vi "Databasetesting.vi"() -> ()   [LabVIEW 2020]
uses:
  Database/Control 1.ctl
  <vilib>/addons/database/Connection.llb/DB Tools Open Connec (Path).vi
  <vilib>/addons/database/_DB Variant To Data/Database Variant To Data.xnode
  <vilib>/addons/database/NI_Database_API.lvlib
panel:
  out "x = y?":bool
  out "number":i32
  out "ID 2":i32 min=0
  in  "stop":bool
  in  "connection information":path=path "C:/Users/User/Documents/Database/Database.udl"
  in  "Tab Control":T1(tab)
  out "Data in Database":string[][][](array[string])
  in  "ID":i32 min=0
  in  "Delete Student":bool
  in  "Add Student":bool
  in  "Add Student Parameters":T2
  in  "Listbox":i32(listbox)
  out "Manipulate Array":string[][](array[string])
  out "Row to Delete":string[][](array[string])
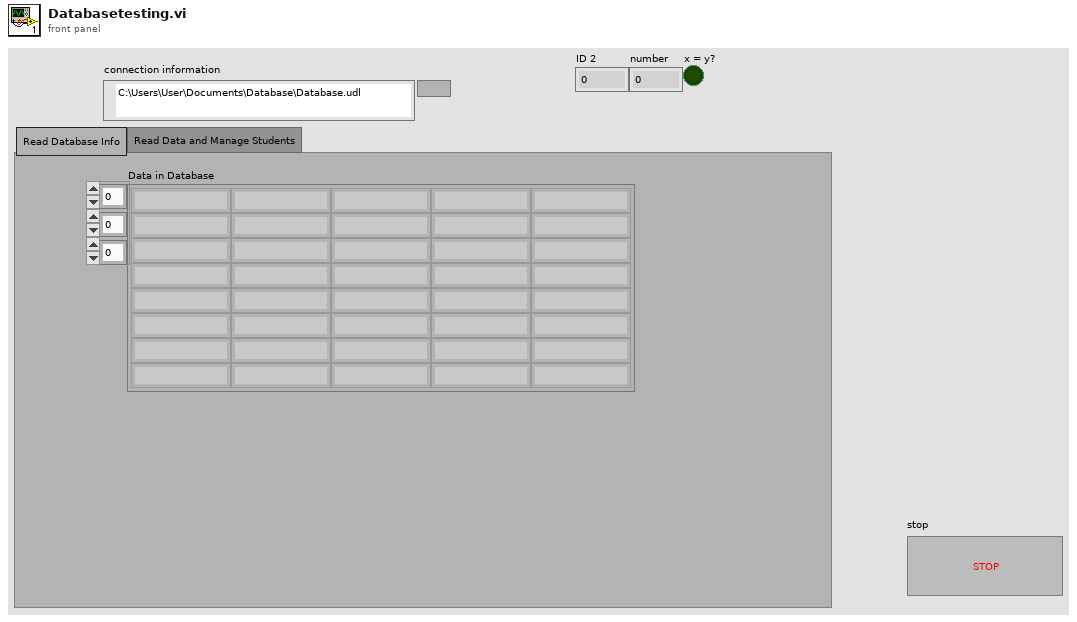
[diagram p1: front panel]
types:
  T1 = enum32{"Read Database Info", "Read Data and Manage Students"}
  T2 = cluster{"Credit Hours":dbl, "Name":string, "Major":string, "Class Rank":string, "ID":i32}
  T3 = typedef "Control 1.ctl" = enum16{"Init Read", "Init Manipulate", "Wait for GUI", "Add Student", "Delete Student", "Stop"}
  T4 = typedef "NI_Database_API.lvlib/Conn ObjectReference.ctl" = refnum<k1>
  T5 = typedef "NI_Database_API.lvlib/DB Tools DataTypes.ctl" = enum16{"String", "Long (I32)", "Single (SGL)", "Double (DBL)", "Date/Time", "Binary"}
  T6 = cluster{"name":string, "database data type":T5, "defined size":i32}[]
  T7 = cluster{"ID":i32, "Name":string, "Major":string, "Credit Hours":dbl, "Class Rank":string}
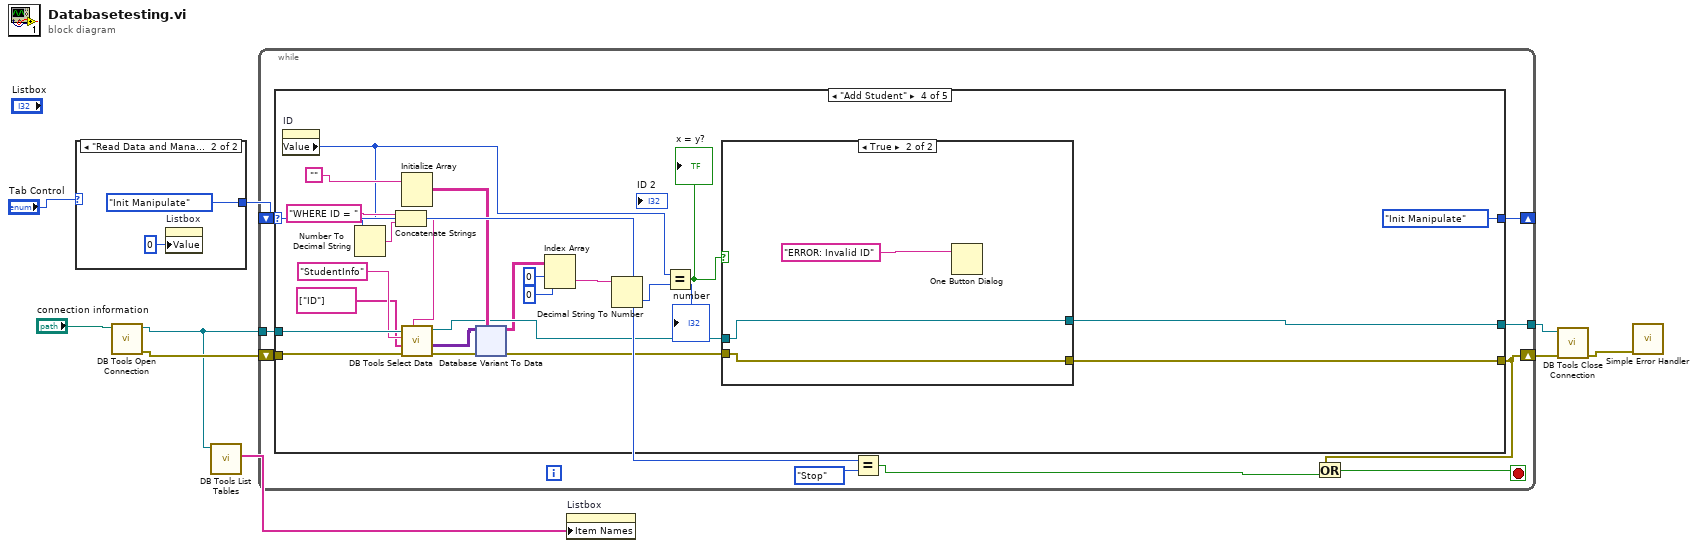
[diagram p0: block diagram]
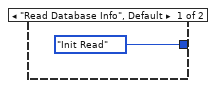
[diagram p2: hidden frame]
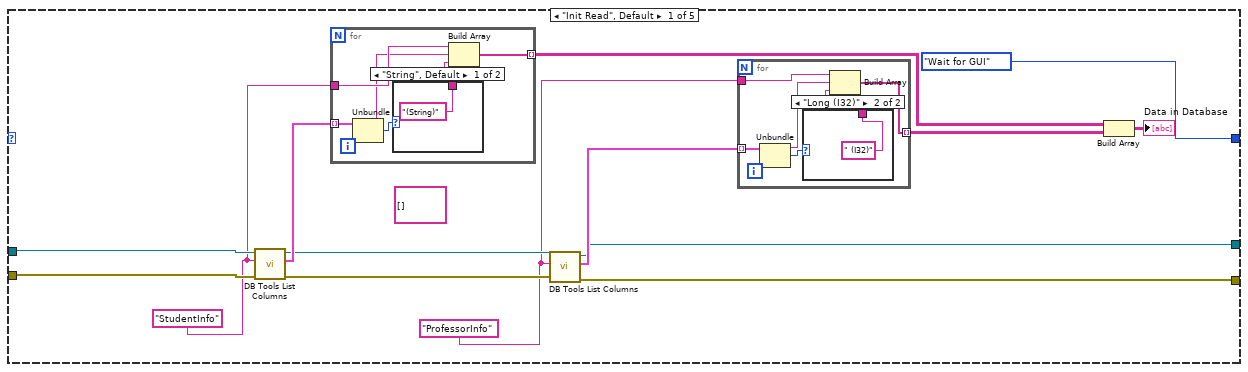
[diagram p3: hidden frame]
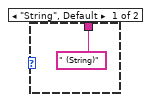
[diagram p4: hidden frame]
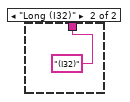
[diagram p5: hidden frame]
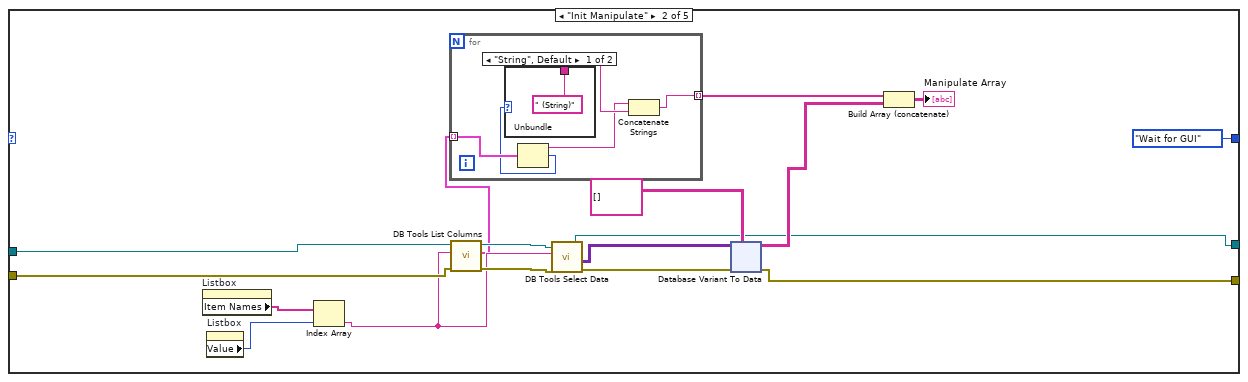
[diagram p6: hidden frame]
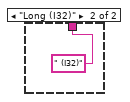
[diagram p7: hidden frame]
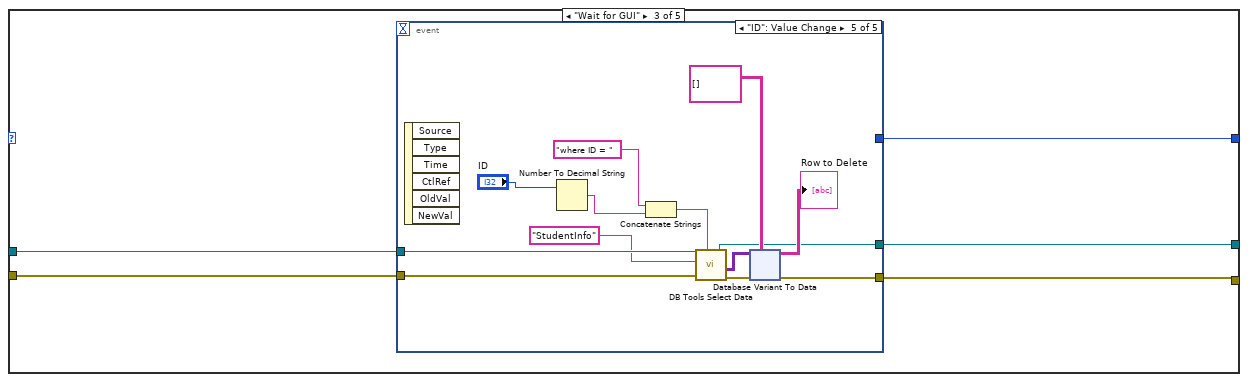
[diagram p8: hidden frame]
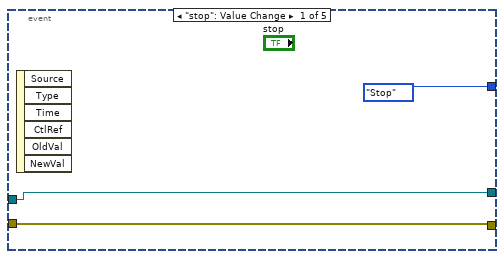
[diagram p9: hidden frame]
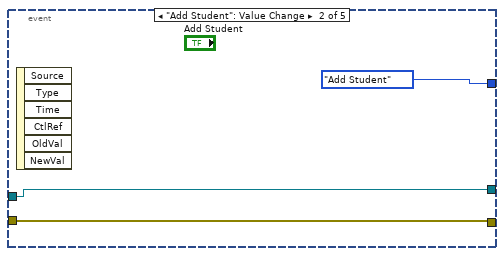
[diagram p10: hidden frame]
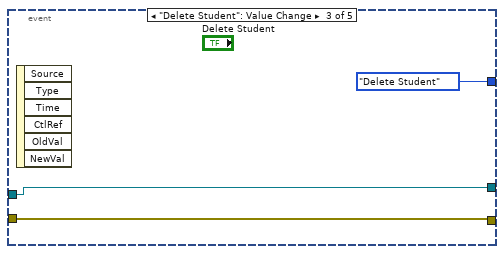
[diagram p11: hidden frame]
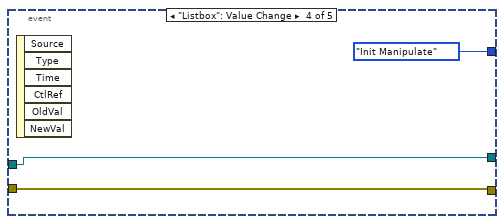
[diagram p12: hidden frame]
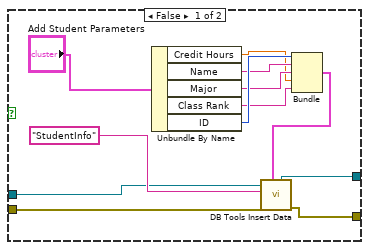
[diagram p13: hidden frame]
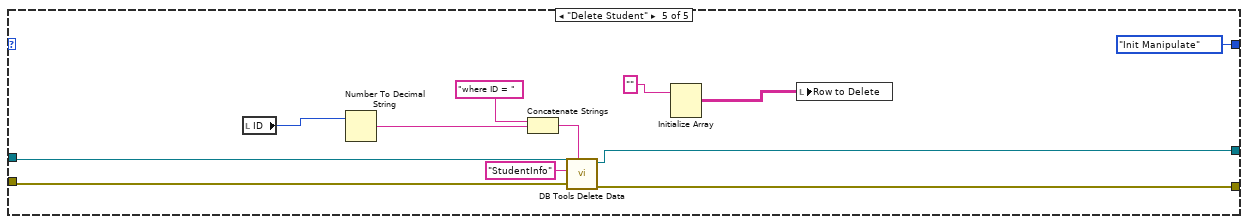
[diagram p14: hidden frame]
diagram:
  n1 = case shown="\"Read Data and Manage Students\"" "Tab Control" {
    tunnel: [Control_1."Init Read" Control_1."Init Manipulate"] -> w7
    frame "Read Database Info", Default {
    }
    frame "Read Data and Manage Students" {
      n2 = property on="Listbox" class="LstBox (strict)"("Value"=0 ("Listbox")) -> ()  [unwired: 2 in, 2 out]
    }
  }
  n3 = call-poly <vilib>:"DB Tools Open Connection.vi"("connection information"="connection information") -> ("error out"=w8:errorcluster, "connection reference"=w6:T4)  [unwired: 7 in]
  n4 = call <vilib>:"DB Tools List Tables.vi"("connection reference"=w6) -> ("tables"=w5:string[])  [unwired: 4 in, 2 out]
  n5 = while {
    tunnel: w6 -> [w19]
    shift-right: [w18] -> _
    shift-left: w7 -> [w21]
    tunnel: [w16] -> w3
    shift-right: [w14] -> w2
    shift-left: w8 -> [w20]
    stop <- w13 stop-if-true
    n6 = case shown="\"Add Student\"" w21 {
      tunnel: w20 -> [w34 w67 w122 w212 w287]
      tunnel: w19 -> [w33 w68 w123 w213 w286]
      tunnel: [Control_1."Wait for GUI" Control_1."Wait for GUI" w124 Control_1."Init Manipulate" Control_1."Init Manipulate"] -> w18
      tunnel: [w28 w54 w121 w216 w285] -> w16
      tunnel: [w27 w53 w120 w214 w284] -> w14
      frame "Init Read", Default {
        w24 = "ProfessorInfo" ("table")
        (unwired) string[][] [] ("initialized array")
        w26 = "StudentInfo" ("table")
        n7 = call <vilib>:"DB Tools List Columns.vi"("error in (no error)"=w34, "table"=w26, "connection reference"=w33) -> ("error out"=w29:errorcluster, "column information"=w32:T6, "connection reference out"=w30:T4)  [unwired: 1 in, 1 out]
        n8 = for {
          tunnel: w32 -> [w49] mode=indexing
          tunnel: w26 -> [w47]
          tunnel: [w44] -> w25 mode=indexing
          n9 = Unbundle(w49) -> ("name"=w46:string, "database data type"=w48:T5)  [unwired: 1 out]
          n10 = case shown="\"String\", Default" w48 {
            tunnel: ["(String)" "(I32)"] -> w45
            frame "String", Default {
            }
            frame "Long (I32)" {
            }
          }
          n11 = Build Array(w47, w46, w45) -> (w44:string[])
        }
        n12 = call <vilib>:"DB Tools List Columns.vi"("error in (no error)"=w29, "table"=w24, "connection reference"=w30) -> ("error out"=w27:errorcluster, "column information"=w31:T6, "connection reference out"=w28:T4)  [unwired: 1 in, 1 out]
        n13 = for {
          tunnel: w31 -> [w41] mode=indexing
          tunnel: w24 -> [w38]
          tunnel: [w36] -> w23 mode=indexing
          n14 = Unbundle(w41) -> ("name"=w39:string, "database data type"=w40:T5)  [unwired: 1 out]
          n15 = case shown="\"Long (I32)\"" w40 {
            tunnel: [" (String)" " (I32)"] -> w37
            frame "String", Default {
            }
            frame "Long (I32)" {
            }
          }
          n16 = Build Array(w38, w39, w37) -> (w36:string[])
        }
        n17 = Build Array(w25, w23) -> (→"Data in Database":string[][][])
      }
      frame "Init Manipulate" {
        n18 = property on="Listbox" class="LstBox (strict)"() -> ("Item Names"=w60:string[])  [unwired: 2 in, 2 out]
        n19 = property on="Listbox" class="LstBox (strict)"() -> ("Value"=w59:i32)  [unwired: 2 in, 2 out]
        n20 = Index Array(array=w60, index=w59) -> (element=w58:string)
        n21 = call <vilib>:"DB Tools List Columns.vi"("error in (no error)"=w67, "table"=w58, "connection reference"=w68) -> ("error out"=w63:errorcluster, "column information"=w57:T6, "connection reference out"=w64:T4)  [unwired: 1 in, 1 out]
        n22 = for {
          tunnel: w57 -> [w73] mode=indexing
          tunnel: [w69] -> w56 mode=indexing
          n23 = Unbundle(w73) -> ("name"=w70:string, "database data type"=w71:T5)  [unwired: 1 out]
          n24 = case shown="\"String\", Default" w71 {
            tunnel: [" (String)" " (I32)"] -> w72
            frame "String", Default {
            }
            frame "Long (I32)" {
            }
          }
          n25 = Concatenate Strings(w70, w72) -> (w69:string)
        }
        n26 = call <vilib>:"DB Tools Select Data.vi"("error in (no error)"=w63, "table"=w58, "connection reference"=w64) -> ("error out"=w65:errorcluster, "data"=w66:variant[][], "connection reference out"=w54:T4)  [unwired: 3 in]
        n27 = xnode "Database Variant To Data"("database variant"=w66, "error in (no error)"=w65, "type"=string[][] [] ("initialized array")) -> ("data"=w61:string[][], "error out"=w53:errorcluster)
        n28 = Build Array (concatenate)(w56, w61) -> (→"Manipulate Array":string[][])
      }
      frame "Wait for GUI" {
        n29 = event shown="[4] \"ID\": Value Change" {
          selector: _ -> [_ _ _ _ _]
          dyn-events: _ -> [_ _ _ _ _]
          timeout: _ -> [_ _ _ _ _]
          tunnel: [Control_1."Stop" Control_1."Add Student" Control_1."Delete Student" Control_1."Init Manipulate" _] -> w124
          tunnel: w123 -> [w126 w129 w132 w135 w148]
          tunnel: w122 -> [w125 w128 w131 w134 w149]
          tunnel: [w126 w129 w132 w135 w137] -> w121
          tunnel: [w125 w128 w131 w134 w138] -> w120
          event "stop": Value Change {
            n30 = event-data() -> ()  [unwired: 1 in, 6 out]
          }
          event "Add Student": Value Change {
            n31 = event-data() -> ()  [unwired: 1 in, 6 out]
          }
          event "Delete Student": Value Change {
            n32 = event-data() -> ()  [unwired: 1 in, 6 out]
          }
          event "Listbox": Value Change {
            n33 = event-data() -> ()  [unwired: 1 in, 6 out]
          }
          event "ID": Value Change {
            n34 = event-data() -> ()  [unwired: 1 in, 6 out]
            n35 = Number To Decimal String(number="ID") -> (decimal integer string=w145:string)  [unwired: 1 in]
            n36 = Concatenate Strings("where ID = " ("string"), w145) -> (w143:string)
            n37 = call <vilib>:"DB Tools Select Data.vi"("condition"=w143, "error in (no error)"=w149, "table"="StudentInfo", "connection reference"=w148) -> ("error out"=w142:errorcluster, "data"=w141:variant[][], "connection reference out"=w137:T4)  [unwired: 2 in]
            n38 = xnode "Database Variant To Data"("database variant"=w141, "error in (no error)"=w142, "type"=string[][] []) -> ("data"=→"Row to Delete":string[][], "error out"=w138:errorcluster)
          }
        }
      }
      frame "Add Student" {
        n39 = property on="ID" class="DigNum (strict)"() -> ("Value"=w194:i32)  [unwired: 2 in, 2 out]
        n40 = Number To Decimal String(number=w194) -> (decimal integer string=w202:string)  [unwired: 1 in]
        n41 = Concatenate Strings("WHERE ID = " ("condition"), w202) -> (w201:string)
        n42 = Initialize Array("") -> (w206:string[][])  [unwired: 2 in]
        n43 = call <vilib>:"DB Tools Select Data.vi"("condition"=w201, "error in (no error)"=w212, "columns"=string[] ["ID"], "table"="StudentInfo", "connection reference"=w213) -> ("error out"=w211:errorcluster, "data"=w210:variant[][], "connection reference out"=w204:T4)  [unwired: 1 in]
        n44 = xnode "Database Variant To Data"("database variant"=w210, "error in (no error)"=w211, "type"=w206) -> ("data"=w200:string[][], "error out"=w205:errorcluster)
        n45 = Index Array(array=w200, index (row)=0, index (col)=0 ("disabled index (col)")) -> (element=w197:string)
        n46 = Decimal String To Number(string=w197) -> (number=w196:i32)  [unwired: 2 in, 1 out]
        "number" <- w196
        n47 = Equal?(x=w194, y=w196) -> (x = y?=w195:bool)
        "x = y?" <- w195
        n48 = case shown="True" w195 {
          tunnel: [w272 w275] -> w216
          tunnel: [w263 w274] -> w214
          tunnel: w205 -> [w262 w274]
          tunnel: w204 -> [w261 w275]
          frame False {
            n49 = Unbundle By Name("Add Student Parameters") -> ("Credit Hours"=w265:dbl, "Name"=w267:string, "Major"=w266:string, "Class Rank"=w264:string, "ID"=w268:i32)
            n50 = Bundle("ID"=w268, "Name"=w267, "Major"=w266, "Credit Hours"=w265, "Class Rank"=w264) -> (w270:T7)  [unwired: 1 in]
            n51 = call <vilib>:"DB Tools Insert Data.vi"("data"=w270, "error in (no error)"=w262, "table"="StudentInfo", "connection reference"=w261) -> ("error out"=w263:errorcluster, "connection reference out"=w272:T4)  [unwired: 6 in]
          }
          frame True {
            n52 = One Button Dialog(message="ERROR: Invalid ID") -> ()  [unwired: 1 in, 1 out]
          }
        }
      }
      frame "Delete Student" {
        n53 = local read "ID"() -> (w282:i32)
        n54 = Number To Decimal String(number=w282) -> (decimal integer string=w281:string)  [unwired: 1 in]
        n55 = Concatenate Strings("where ID = ", w281) -> (w279:string)
        n56 = call <vilib>:"DB Tools Delete Data.vi"("condition"=w279, "error in (no error)"=w287, "table"="StudentInfo", "connection reference"=w286) -> ("error out"=w284:errorcluster, "connection reference out"=w285:T4)  [unwired: 6 in]
        n57 = Initialize Array("") -> (w276:string[][])  [unwired: 2 in]
        n58 = local write "Row to Delete"(w276) -> ()
      }
    }
    n59 = Equal?(x=w21, y=Control_1."Stop") -> (x = y?=w15:bool)
    n60 = Or(x=w14, y=w15) -> (x .or. y?=w13:bool)
  }
  n61 = property on="Listbox" class="LstBox (strict)"("Item Names"=w5) -> ()  [unwired: 2 in, 2 out]
  n62 = call <vilib>:"DB Tools Close Connection.vi"("error in (no error)"=w2, "connection reference"=w3) -> ("error out"=w1:errorcluster)  [unwired: 5 in]
  n63 = call <vilib>:"Simple Error Handler.vi"("error in (no error)"=w1) -> ()  [unwired: 4 in, 5 out]
